vi "Import_Clipboard.vi"(8 "error in (no error)":errorcluster {"code" min=0 max=0}, 10 "Picture in":picture) -> (0 "error out":errorcluster {"code" min=0 max=0}, 1 "Valid?":bool, 2 "Picture":picture)   [LabVIEW 2020]
uses:
  <vilib>/picture/picture.llb/imagedata.ctl
  vi.lib/LabVIEW Icon API/lv_icon/lv_icon.lvlib
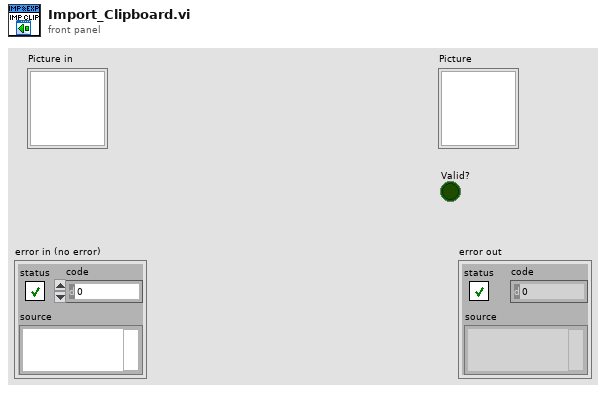
[diagram p1: front panel]
types:
  T1 = typedef "imagedata.ctl" = cluster{"image type":i32, "image depth":i32, "image":u8[], "mask":u8[], "colors":u32[], "Rectangle":cluster{"left":i16, "top":i16, "right":i16, "bottom":i16}}
  T2 = typedef "LVRectTypeDef.ctl" = cluster{"left":i16, "top":i16, "right":i16, "bottom":i16}
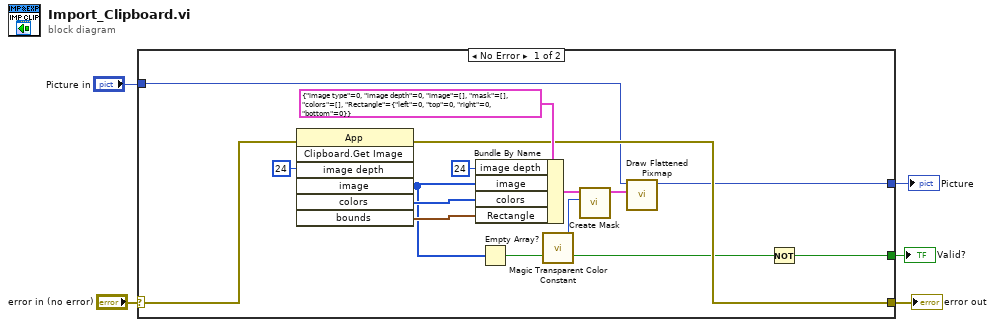
[diagram p0: block diagram]
diagram:
  n1 = case shown="No Error" "error in (no error)" {
    selector: "error in (no error)" -> [w13 w21]
    tunnel: [w12 w21] -> w4
    tunnel: [w11 _] -> w3
    tunnel: "Picture in" -> [w10 _]
    tunnel: [w7 _] -> w1
    frame No Error {
      n2 = invoke class="App" method="Clipboard.Get Image"(error in=w13, "image depth"=24 ("Image Depth")) -> (error out=w12:errorcluster, "image"=w9:u8[], "colors"=w17:u32[], "bounds"=w18:T2)  [unwired: 5 in, 3 out]
      n3 = Bundle By Name(cluster=T1 {"image type"=0, "image depth"=0, "image"=[], "mask"=[], "colors"=[], "Rectangle"={"left"=0, "top"=0, "right"=0, "bottom"=0}} ("image data"), "image depth"=24, "image"=w9, "colors"=w17, "Rectangle"=w18) -> (w15:T1)
      n4 = Empty Array?(array=w9) -> (empty?=w8:bool)
      n5 = call "Magic Transparent Color Constant.vi"() -> ("Magic transparent color constant"=w6:u32)  [unwired: 11 out]
      n6 = call <vilib>:"Create Mask.vi"("Mask Color (Black)"=w6, "image data"=w15) -> ("image data"=w14:T1)  [unwired: 2 in, 7 out]
      n7 = call <vilib>:"Draw Flattened Pixmap.vi"("image data"=w14, "picture"=w10) -> ("new picture"=w11:picture)  [unwired: 7 out]
      n8 = Not(x=w8) -> (.not. x?=w7:bool)
    }
    frame Error {
    }
  }
  "error out" <- w4
  "Picture" <- w3
  "Valid?" <- w1
